vi "fr string to dbl small.vi"(7 "String":string) -> (8 "number":dbl)   [LabVIEW 2018]
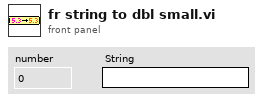
[diagram p1: front panel]
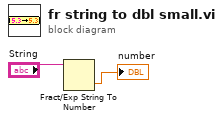
[diagram p0: block diagram]
diagram:
  n1 = Fract/Exp String To Number(string="String") -> (number=→"number":dbl)  [unwired: 3 in, 1 out]
